vi "Comm String Send Command.vi"(0 "niDTS Comm EXE in":refnum<class "niDTS Comm EXE.lvclass">, 5 "Command":string, 7 "Args":string, 11 "error in (no error)":errorcluster) -> (4 "niDTS Comm EXE out":refnum<class "niDTS Comm EXE.lvclass">, 6 "Response":string, 15 "error out":errorcluster)   [LabVIEW 2015, in "niDTS CommLib.lvlib" / "niDTS Comm EXE.lvclass"]
uses:
  niDTS Comm EXE.lvclass
  niDTS Comm EXE.lvclass/niDTS Comm EXE.ctl
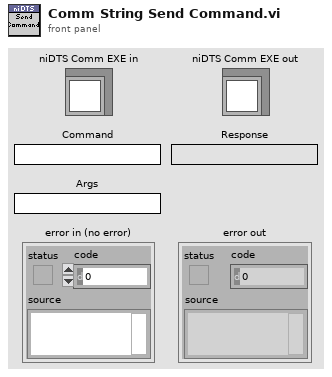
[diagram p1: front panel]
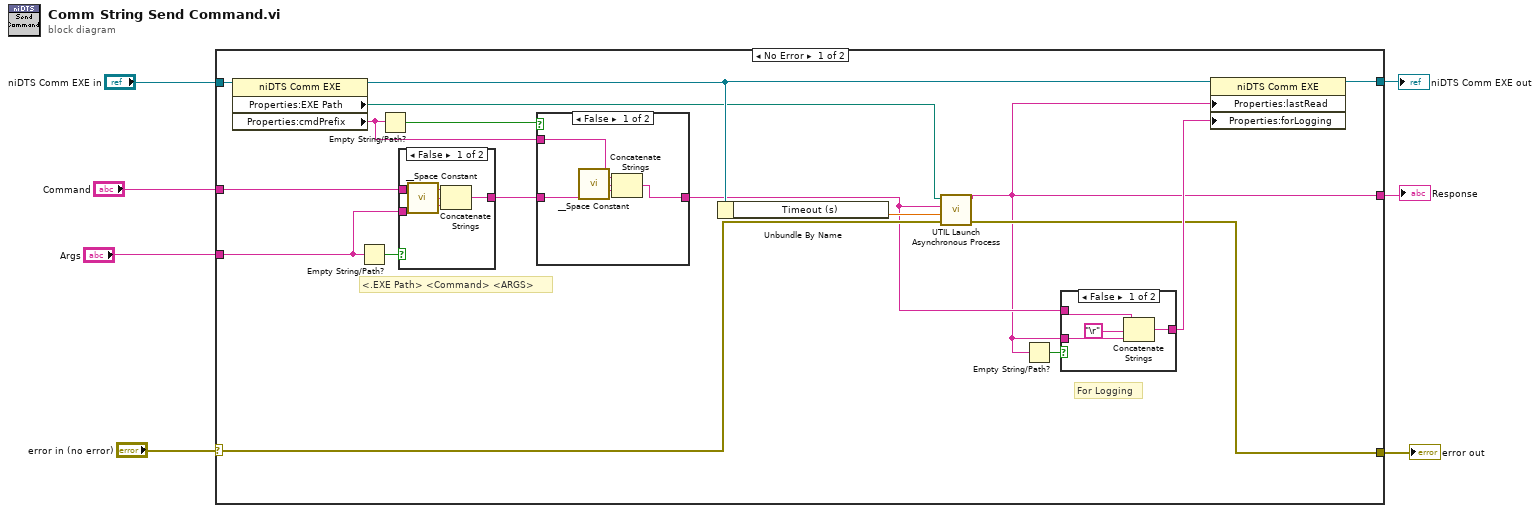
[diagram p0: block diagram]
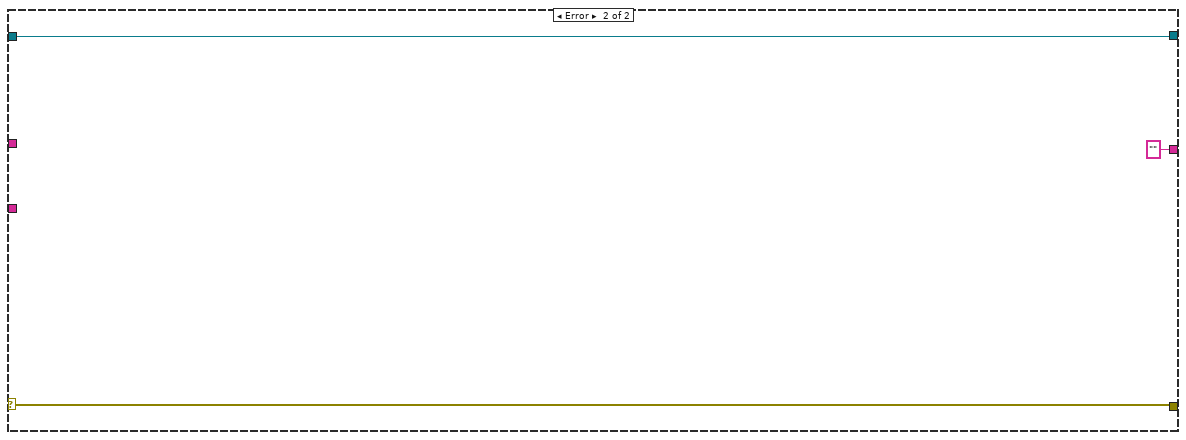
[diagram p5: hidden frame]
diagram:
  n1 = case shown="No Error" "error in (no error)" {
    selector: "error in (no error)" -> [w17 w42]
    tunnel: "niDTS Comm EXE in" -> [w19 w40]
    tunnel: "Command" -> [w13 _]
    tunnel: "Args" -> [w23 _]
    tunnel: [w21 w40] -> w2
    tunnel: [w8 "" ("standard output")] -> w3
    tunnel: [w16 w42] -> w1
    frame No Error {
      # "For Logging"
      # "<.EXE Path> <Command> <ARGS>"
      n2 = property class="niDTS Comm EXE"(reference=w19) -> (reference out=w18:refnum<class "niDTS Comm EXE.lvclass">, "Properties:EXE Path"=w14:path, "Properties:cmdPrefix"=w10:string)  [unwired: 1 in, 1 out]
      n3 = Empty String/Path?(string/path=w23) -> (empty?=w24:bool)
      n4 = Empty String/Path?(string/path=w10) -> (empty?=w12:bool)
      n5 = case shown="False" w24 {
        tunnel: w13 -> [w38 w39]
        tunnel: [w35 w39] -> w11
        tunnel: w23 -> [w36 _]
        frame False {
          n6 = call "__Space Constant.vi"() -> ("String"=w37:string)
          n7 = Concatenate Strings(w38, w37, w36) -> (w35:string)
        }
        frame True {
        }
      }
      n8 = case shown="False" w12 {
        tunnel: w11 -> [w27 w29]
        tunnel: [w25 w29] -> w9
        tunnel: w10 -> [w26 _]
        frame False {
          n9 = call "__Space Constant.vi"() -> ("String"=w28:string)
          n10 = Concatenate Strings(w26, w28, w27) -> (w25:string)
        }
        frame True {
        }
      }
      n11 = Unbundle By Name(w18) -> ("Timeout (s)"=w15:dbl)
      n12 = call "UTIL Launch Asynchronous Process.vi"("error in (no error)"=w17, "Timeout (5s)"=w15, "Arguments"=w9, "Process Path"=w14) -> ("error out"=w16:errorcluster, "Standard Output"=w8:string)  [unwired: 6 in]
      n13 = Empty String/Path?(string/path=w8) -> (empty?=w22:bool)
      n14 = case shown="False" w22 {
        tunnel: [w32 w34] -> w20
        tunnel: w9 -> [w31 w34]
        tunnel: w8 -> [w30 _]
        frame False {
          n15 = Concatenate Strings(w31, "\r", w30) -> (w32:string)
        }
        frame True {
        }
      }
      n16 = property class="niDTS Comm EXE"(reference=w18, "Properties:lastRead"=w8, "Properties:forLogging"=w20) -> (reference out=w21:refnum<class "niDTS Comm EXE.lvclass">)  [unwired: 1 in, 1 out]
    }
    frame Error {
    }
  }
  "error out" <- w1
  "niDTS Comm EXE out" <- w2
  "Response" <- w3
